vi "ex_5.vi"() -> ()   [LabVIEW 2020]
panel:
  out "Numeric":i32
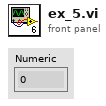
[diagram p1: front panel]
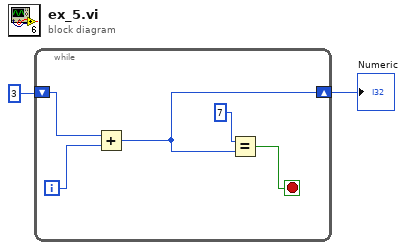
[diagram p0: block diagram]
diagram:
  n1 = while {
    shift-right: [w3] -> w1
    shift-left: 3 -> [w7]
    i -> [w6]
    stop <- w5 stop-if-true
    n2 = Add(x=w7, y=w6) -> (x+y=w3:i32)
    n3 = Equal?(x=7, y=w3) -> (x = y?=w5:bool)
  }
  "Numeric" <- w1
